vi "Close.vi"(8 "error in (no error)":errorcluster, 11 "Data.PG in":refnum<class "LV-Data.PGSQL.lvclass">) -> (0 "error out":errorcluster, 3 "Data.PG out":refnum<class "LV-Data.PGSQL.lvclass">)   [LabVIEW 2019, in "LV-Data.PGSQL.lvclass"]
uses:
  LV-Data.PGSQL.lvclass
  <vilib>/JDP Science/PostgreSQL Library/Connection/PQ Connection.lvclass
  LV-Data.PGSQL.lvclass/LV-Data.PGSQL.ctl
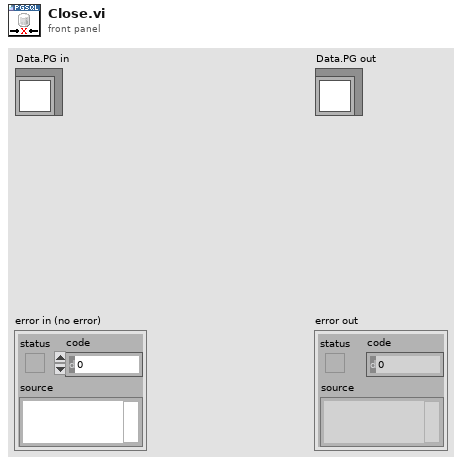
[diagram p1: front panel]
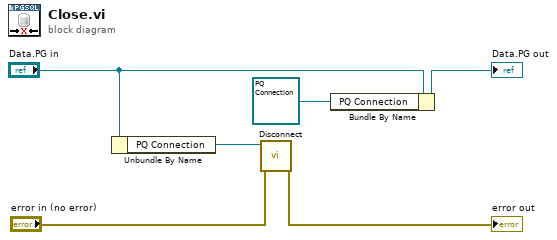
[diagram p0: block diagram]
diagram:
  n1 = Unbundle By Name("Data.PG in") -> ("PQ Connection"=w2:refnum<class "PQ Connection.lvclass">)
  n2 = call <vilib>:"Disconnect.vi"("error in (no error)"="error in (no error)", "PQ Connection in"=w2) -> ("error out"=→"error out":errorcluster)  [unwired: 9 in]
  n3 = Bundle By Name(cluster="Data.PG in", "PQ Connection"=refnum<class "PQ Connection.lvclass"> refnum) -> (→"Data.PG out":refnum<class "LV-Data.PGSQL.lvclass">)
